vi "GetDeviceParameterValue.vi"(8 "error in":errorcluster, 9 "Parameter Name":string, 10 "Device Command":string, 11 "connection ID in":refnum<k5>) -> (0 "error out":errorcluster, 1 "Error Info":T1, 2 "Parameter":cluster{"Name":string, "Value":string}, 3 "connection ID out":refnum<k5>, 4 "Log String":string, 5 "OK":bool)   [LabVIEW 2020, in "ProdigyRemoteControl.lvlib"]
uses:
  ProdigyRemoteControl.lvlib
  DEFINITIONS/DEF_RcError.ctl
  DEFINITIONS/DEF_RcCmd.ctl
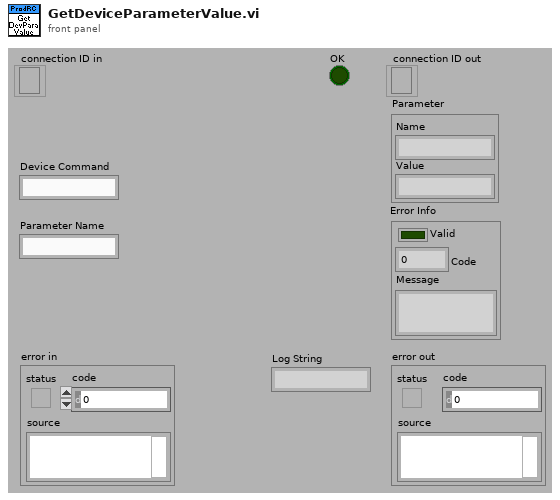
[diagram p1: front panel]
types:
  T1 = typedef "ProdigyRemoteControl.lvlib/DEF_RcError.ctl" = cluster{"Valid":bool, "Code":u16, "Message":string}
  T2 = typedef "ProdigyRemoteControl.lvlib/DEF_RcCmd.ctl" = string
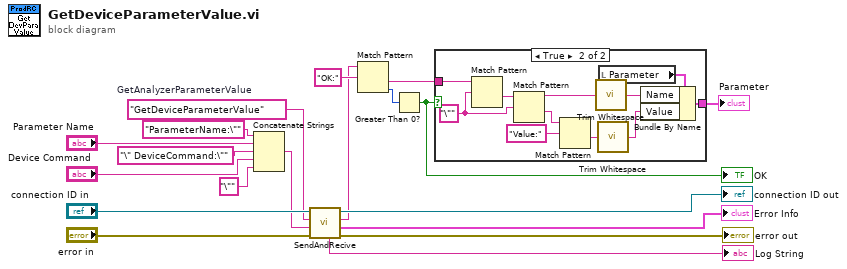
[diagram p0: block diagram]
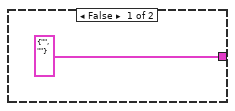
[diagram p2: hidden frame]
diagram:
  w15 = T2 "GetDeviceParameterValue"  # GetAnalyzerParameterValue
  n1 = Concatenate Strings("ParameterName:\"" ("string"), "Parameter Name", "\" DeviceCommand:\"" ("string"), "Device Command", "\"" ("string")) -> (w10:string)
  n2 = call "SendAndRecive.vi"("error in"="error in", "Parameters"=w10, "Command"=w15, "connection ID in"="connection ID in") -> ("error out"=→"error out":errorcluster, "Error Info"=→"Error Info":T1, "Answer"=w8:string, "connection ID out"=→"connection ID out":refnum<k5>, "Log String"=→"Log String":string)  [unwired: 3 in]
  n3 = Match Pattern(string=w8, regular expression="OK:") -> (after substring=w5:string, offset past match=w7:i32)  [unwired: 1 in, 2 out]
  n4 = Greater Than 0?(x=w7) -> (x > 0?=w4:bool)
  "OK" <- w4
  n5 = case shown="True" w4 {
    tunnel: [cluster{"Name":string, "Value":string} {"Name"="", "Value"=""} ("Parameter") w22] -> w6
    tunnel: w5 -> [_ w21]
    frame False {
    }
    frame True {
      w28 = "\"" ("regular expression")
      n6 = Match Pattern(string=w21, regular expression=w28) -> (after substring=w29:string)  [unwired: 1 in, 3 out]
      n7 = Match Pattern(string=w29, regular expression=w28) -> (before substring=w26:string, after substring=w27:string)  [unwired: 1 in, 2 out]
      n8 = Match Pattern(string=w27, regular expression="Value:") -> (after substring=w30:string)  [unwired: 1 in, 3 out]
      n9 = call <vilib>:"Trim Whitespace.vi"("string"=w26) -> ("trimmed string"=w24:string)  [unwired: 1 in]
      n10 = call <vilib>:"Trim Whitespace.vi"("string"=w30) -> ("trimmed string"=w23:string)  [unwired: 1 in]
      n11 = local read "Parameter"() -> (w25:cluster{"Name":string, "Value":string})
      n12 = Bundle By Name(cluster=w25, "Name"=w24, "Value"=w23) -> (w22:cluster{"Name":string, "Value":string})
    }
  }
  "Parameter" <- w6
